vi "Util_FP Control.vi"(8 "error in (no error)":errorcluster, 11 "Function":T1) -> (0 "error out":errorcluster)   [LabVIEW 2020]
uses:
  FP Control Functions.ctl
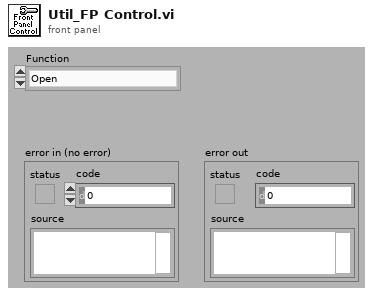
[diagram p1: front panel]
types:
  T1 = typedef "FP Control Functions.ctl" = enum16{"Open", "Close", "Bring To Front", "Center"}
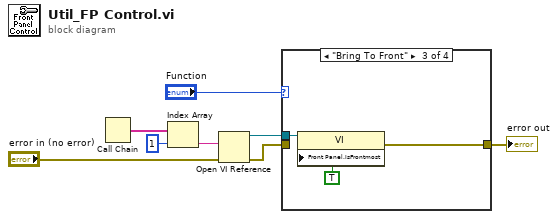
[diagram p0: block diagram]
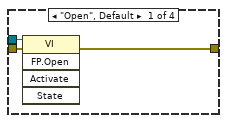
[diagram p2: hidden frame]
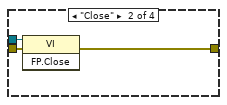
[diagram p3: hidden frame]
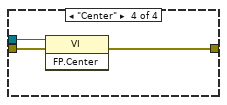
[diagram p4: hidden frame]
diagram:
  n1 = Call Chain() -> (call chain=w5:string[])
  n2 = Index Array(array=w5, index=1) -> (element=w3:string)
  n3 = Open VI Reference(vi path=w3, error in (no error)="error in (no error)") -> (vi reference=w7:refnum<vi>, error out=w8:errorcluster)  [unwired: 1 in, 3 out]
  n4 = case shown="\"Bring To Front\"" "Function" {
    tunnel: w8 -> [w11 w14 _ w19]
    tunnel: w7 -> [w10 w13 w17 w20]
    tunnel: [w9 w12 w15 w18] -> w1
    frame "Open", Default {
      n5 = invoke class="VI" method="FP.Open"(reference=w10, error in=w11) -> (error out=w9:errorcluster)  [unwired: 3 in, 4 out]
    }
    frame "Close" {
      n6 = invoke class="VI" method="FP.Close"(reference=w13, error in=w14) -> (error out=w12:errorcluster)  [unwired: 1 in, 2 out]
    }
    frame "Bring To Front" {
      n7 = property class="VI"(reference=w17, "Front Panel.IsFrontmost"=TRUE) -> (error out=w15:errorcluster)  [unwired: 1 in, 1 out]
    }
    frame "Center" {
      n8 = invoke class="VI" method="FP.Center"(reference=w20, error in=w19) -> (error out=w18:errorcluster)  [unwired: 1 in, 2 out]
    }
  }
  "error out" <- w1
